vi "Error Sender.vi"   [LabVIEW 2012]
uses:
  controls/Error Sender Enum.ctl
types:
  T1 = typedef "Error Sender Enum.ctl" = enum16{"Initialize", "Listen for Reader", "Send Error Messages"}
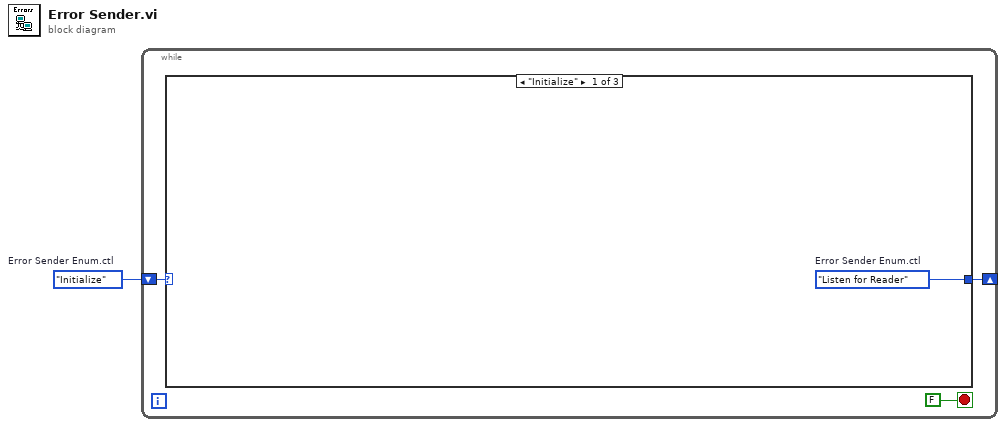
[diagram p0: block diagram]
diagram:
  w1 = Error_Sender_Enum."Initialize"  # Error Sender Enum.ctl
  n1 = while {
    shift-right: [w4] -> _
    shift-left: w1 -> [w3]
    stop <- FALSE stop-if-true
    n2 = case shown="\"Initialize\"" w3 {
      tunnel: [w5 _ _] -> w4
      frame "Initialize" {
        w5 = Error_Sender_Enum."Listen for Reader"  # Error Sender Enum.ctl
      }
      frame "Listen for Reader" {
      }
      frame "Send Error Messages" {
      }
    }
  }
